vi "SPECTRUM Set Settings_corrected.vi"(0 "span":dbl, 1 "rbw":dbl, 2 "enableVBW":bool, 3 "vbw":dbl, 4 "traceLength":i32, 5 "window":u32(ring) items=["SpectrumWindow_Kaiser", "SpectrumWindow_Mil6dB", "SpectrumWindow_BlackmanHarris", "SpectrumWindow_Rectangle", "SpectrumWindow_FlatTop", "SpectrumWindow_Hann"], 6 "verticalUnit":u32(ring) items=["SpectrumVerticalUnit_dBm", "SpectrumVerticalUnit_Watt", "SpectrumVerticalUnit_Volt", "SpectrumVerticalUnit_Amp", "SpectrumVerticalUnit_dBmV"], 7 "error in (no error)":errorcluster) -> (20 "function return":u32(ring), 27 "error out":errorcluster)   [LabVIEW 2017, in "RSA_API.lvlib"]
doc: "RSA_API_DLL ReturnStatus SPECTRUM_SetSettings(Spectrum_Settings settings);"
uses:
  <userlib>/RSA_API/RSA_API.lvlib
  Tektronix/RSA_API/lib/x86/RSA_API.dll
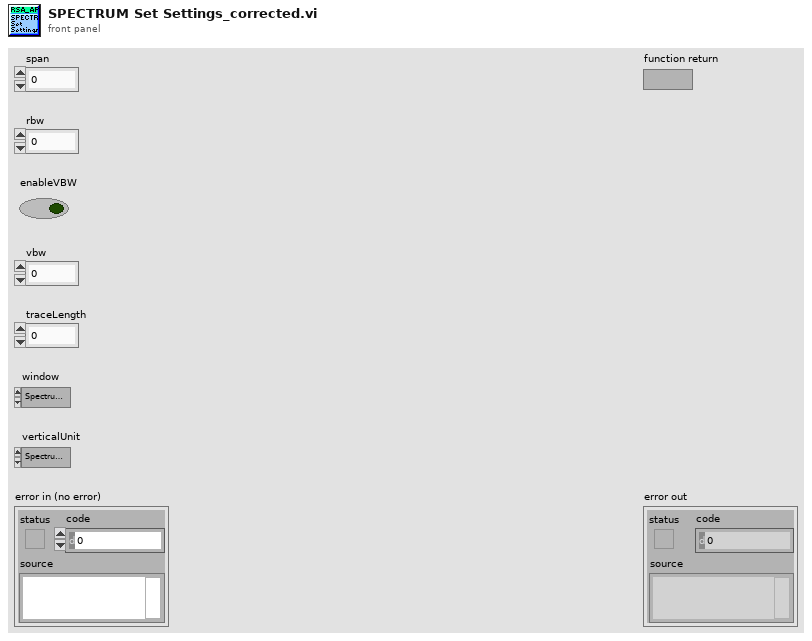
[diagram p1: front panel]
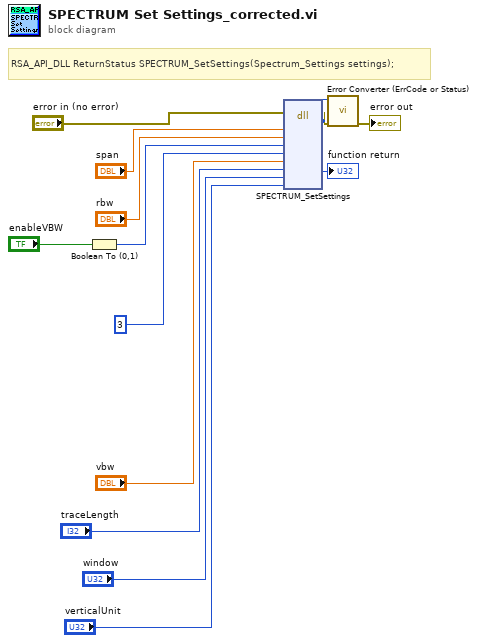
[diagram p0: block diagram]
diagram:
  # "RSA_API_DLL ReturnStatus SPECTRUM_SetSettings(Spectrum_Settings settings);"
  n1 = Boolean To (0,1)(Boolean="enableVBW") -> (0, 1=w9:i16)
  n2 = dll-call lib="C:/Tektronix/RSA_API/lib/x86/RSA_API.*" fn="SPECTRUM_SetSettings"(error in="error in (no error)", "span"="span", "rbw"="rbw", "enableVBW"=w9, "@dummy control@"=i8 3, "vbw"="vbw", "traceLength"="traceLength", "window"="window", "verticalUnit"="verticalUnit") -> (error out=w2:errorcluster, "return type"=w13:u32)  [unwired: 10 in, 1 out]
  "function return" <- w13
  n3 = call <userlib>:"Error Converter (ErrCode or Status).vi"("error in (no error)"=w2, "error code"=w13) -> ("error out"=→"error out":errorcluster)  [unwired: 9 in]
